vi "_TangoToLabviewError.vi"(1 "location":string="[unknown location]", 2 "error stack":string[](array[string])=["unknown error", "Unknown Error", "Unknown Error", "Unknown Error"], 3 "error code":i32=-1) -> (0 "error out":errorcluster)   [LabVIEW 2014, in "tango.lvlib"]
uses:
  tango.lvlib
panel:
  # "This Vi is deprecated and only maintained for backward compatibility. Please use  _TangoExceptionToLabviewError instead."
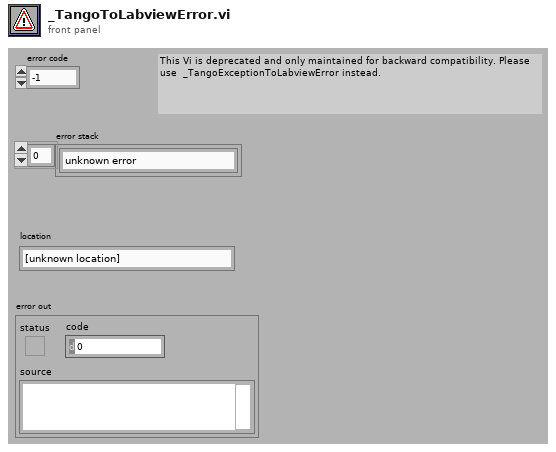
[diagram p1: front panel]
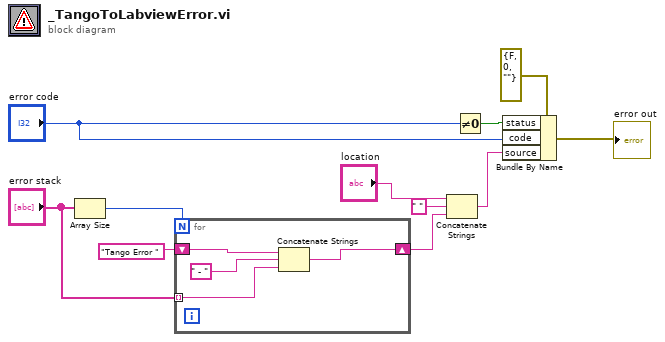
[diagram p0: block diagram]
diagram:
  n1 = Array Size(array="error stack") -> (size(s)=w11:i32)
  n2 = for {
    N: w11 -> [_]
    tunnel: "error stack" -> [w14] mode=indexing
    shift-right: [w12] -> w4
    shift-left: "Tango Error " -> [w15]
    n3 = Concatenate Strings(w15, " - " ("string"), w14) -> (w12:string)
  }
  n4 = Concatenate Strings("location", " " ("string"), w4) -> (w3:string)
  n5 = Not Equal To 0?(x="error code") -> (x != 0?=w2:bool)
  n6 = Bundle By Name(cluster=errorcluster {"status"=FALSE, "code"=0, "source"=""} ("error out"), "status"=w2, "code"="error code", "source"=w3) -> (→"error out":errorcluster)
